vi "Remove Alias If Valid.vi"(8 "error in (no error)":errorcluster, 10 "Alias":string, 11 "Aliases Ref in":T1 format="%.0x") -> (0 "error out":errorcluster, 3 "Aliases Ref out":T1 format="%.0x")   [LabVIEW 2020, in "Routing and Faulting System Explorer.lvlib"]
uses:
  Routing and Faulting System Explorer.lvlib
  <vilib>/NI VeriStand/Custom Device API/Custom Device Item Ref.ctl
  Scripting/Routing and Faulting Scripting.lvlib
  <vilib>/NI VeriStand/Custom Device API/Custom Device API.lvlib
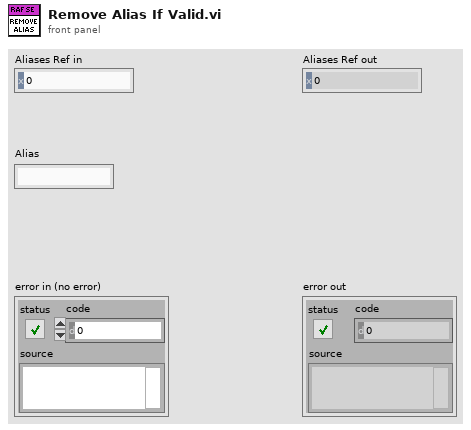
[diagram p1: front panel]
types:
  T1 = typedef "Custom Device API.lvlib/Custom Device Item Ref.ctl" = u64
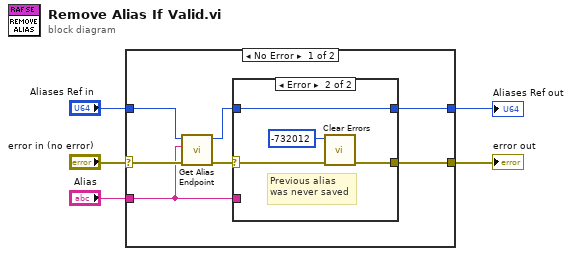
[diagram p0: block diagram]
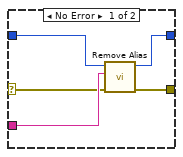
[diagram p2: hidden frame]
diagram:
  n1 = case shown="No Error" "error in (no error)" {
    selector: "error in (no error)" -> [w9 w22]
    tunnel: "Aliases Ref in" -> [w10 w23]
    tunnel: "Alias" -> [w6 _]
    tunnel: [w8 w23] -> w1
    tunnel: [w7 w22] -> w2
    frame No Error {
      n2 = call "Get Alias Endpoint.vi"("error in"=w9, "alias"=w6, "endpoint aliases in"=w10) -> ("error out"=w11:errorcluster, "endpoint aliases out"=w12:T1)  [unwired: 6 in, 1 out]
      n3 = case shown="Error" w11 {
        selector: w11 -> [w15 w20]
        tunnel: w12 -> [w17 w21]
        tunnel: w6 -> [w16 _]
        tunnel: [w13 w21] -> w8
        tunnel: [w14 w19] -> w7
        frame No Error {
          n4 = call "Remove Alias.vi"("error in"=w15, "alias"=w16, "endpoint aliases in"=w17) -> ("error out"=w14:errorcluster, "endpoint aliases out"=w13:T1)  [unwired: 7 in]
        }
        frame Error {
          # "Previous alias\nwas never saved"
          n5 = call <vilib>:"Clear Errors.vi"("error in (no error)"=w20, "specific error code to clear (0: all)"=-732012) -> ("error out"=w19:errorcluster)  [unwired: 4 in, 1 out]
        }
      }
    }
    frame Error {
    }
  }
  "error out" <- w2
  "Aliases Ref out" <- w1
